vi "VIPM package Testing automation - runner.vi"(8 "error in (no error)":errorcluster, 11 "Project Refnum":refnum<vi>) -> (0 "error out":errorcluster, 3 "Test Suite Results":refnum<class "Test Result.lvclass">)   [LabVIEW 2016]
uses:
  <vilib>/addons/_JKI Toolkits/Caraya/classes/Test Result/Test Result.lvclass
  <vilib>/addons/_JKI Toolkits/Caraya/classes/Test Runner/Test Runner.lvclass/Test Runner.ctl
  <vilib>/addons/_JKI Toolkits/Caraya/classes/Test Report.JUnit/Test Report.JUnit.lvclass
  C:/Program Files (x86)/National Instruments/LabVIEW 2016/vi.lib/addons/_JKI Toolkits/Caraya/classes/Test Report/Test Report.lvclass
  <vilib>/addons/_JKI Toolkits/Caraya/classes/Test Runner.Project/Test Runner.Project.lvclass
  C:/Program Files (x86)/National Instruments/LabVIEW 2016/vi.lib/addons/_JKI Toolkits/Caraya/classes/Test Runner/Test Runner.lvclass
  <vilib>/addons/_JKI Toolkits/Caraya/classes/Test Suite/Define Test Suite (Default).vi
  <vilib>/addons/_JKI Toolkits/Caraya/classes/Test Suite/Test Suite.lvclass
  <vilib>/addons/_JKI Toolkits/Caraya/classes/Test Runner/Test Runner.lvclass
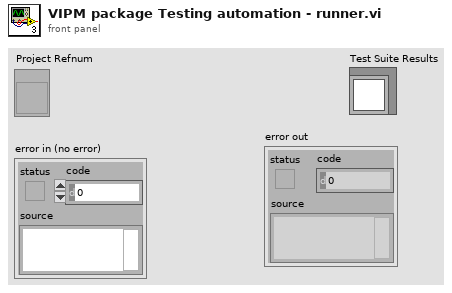
[diagram p1: front panel]
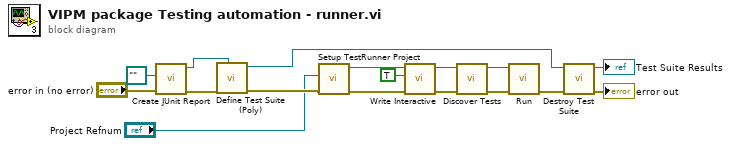
[diagram p0: block diagram]
diagram:
  n1 = call <vilib>:"Create JUnit Report.vi"("error in (no error)"="error in (no error)", "Report Path"=path "") -> ("error out"=w8:errorcluster, "Test Report.JUnit out"=w7:refnum<class "Test Report.JUnit.lvclass">)  [unwired: 8 in]
  n2 = call-poly <vilib>:"Define Test Suite (Poly).vi"("Test Report (optional)"=w7, "error in (no error)"=w8) -> ("error out"=w6:errorcluster, "Test Suite"=w9:refnum<class "Test Suite.lvclass">)  [unwired: 7 in, 1 out]
  n3 = call <vilib>:"Setup TestRunner Project.vi"("error in (no error)"=w6, "Project Refnum"="Project Refnum") -> ("error out"=w16:errorcluster, "Test Runner.Project out"=w14:refnum<class "Test Runner.Project.lvclass">)  [unwired: 8 in]
  n4 = call <vilib>:"Write Interactive.vi"("Interactive"=TRUE, "Test Runner in"=w14) -> ("Test Runner out"=w13:refnum<class "Test Runner.Project.lvclass">)  [unwired: 9 in]
  n5 = call <vilib>:"Discover Tests.vi"("error in (no error)"=w16, "Test Runner in"=w13) -> ("error out"=w11:errorcluster, "Test Runner out"=w12:refnum<class "Test Runner.Project.lvclass">)  [unwired: 8 in]
  n6 = call <vilib>:"Run.vi"("error in (no error)"=w11, "Test Runner in"=w12) -> ("error out"=w10:errorcluster)  [unwired: 7 in, 2 out]
  n7 = call-dynamic "Destroy Test Suite.vi"("error in (no error)"=w10, "Test Suite in"=w9) -> ("error out"=→"error out":errorcluster, "Test Suite Results"=→"Test Suite Results":refnum<class "Test Result.lvclass">)  [unwired: 8 in]
